vi "GetData.vi"(8 "error in (no error)":errorcluster, 10 "Channel":u8, 11 "ID In":i32) -> (0 "error out":errorcluster, 1 "Data information":T2 {"NbCols" min=5 max=7}, 2 "Current values":T1 {"EceRangeMax" format="%.2e"; "EceRangeMin" format="%.2e"; "EweRangeMax" format="%.2e"; "EweRangeMin" format="%.2e"; "Ece" format="%.2e"; "Ewe" format="%.2e"; "I" format="%.2e"; "TimeBase" format="%.2e"}, 3 "ID Out":i32, 4 "row2":u32[](array[numeric]), 5 "Data":dbl[][](array[numeric]), 6 "row3":u32[](array[numeric]), 7 "row4":u32[](array[numeric]))   [LabVIEW 2022 SP3, in "EClib functions.lvlib"]
doc: "Gets data from the selected channel."
uses:
  EClib functions.lvlib
  daff55f7-81b9-4493-b743-378d3d3ed068.vi
  68c41494-4949-413e-9d31-4f27a4ef7998.vi
  99021f18-7fd7-4697-be58-36819a2c27f0.vi
  61984fb0-cc5b-45ed-9757-d3fa5cda0840.vi
  fc0931df-71c6-4ee7-b843-224dab94ccff.vi
  daff55f7-81b9-4493-b743-378d3d3ed068.vi/7c5cbe08-cd9e-464e-aac1-cffdf31a2600.vi
  68c41494-4949-413e-9d31-4f27a4ef7998.vi/7c5cbe08-cd9e-464e-aac1-cffdf31a2600.vi
  99021f18-7fd7-4697-be58-36819a2c27f0.vi/db331072-caa1-433a-9332-c619978f86e3.vi
  61984fb0-cc5b-45ed-9757-d3fa5cda0840.vi/7c5cbe08-cd9e-464e-aac1-cffdf31a2600.vi
  fc0931df-71c6-4ee7-b843-224dab94ccff.vi/7c5cbe08-cd9e-464e-aac1-cffdf31a2600.vi
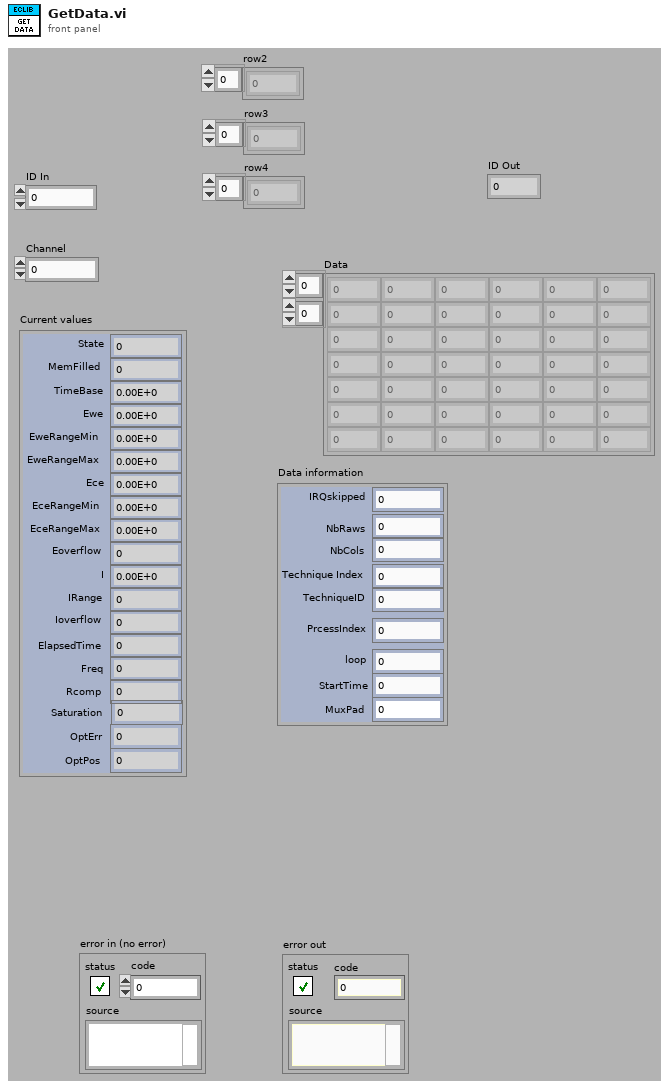
[diagram p1: front panel]
types:
  T1 = cluster{"State":i32, "MemFilled":i32, "TimeBase":sgl, " Ewe":sgl, " EweRangeMin":sgl, " EweRangeMax":sgl, "Ece":sgl, "EceRangeMin":sgl, "EceRangeMax":sgl, "Eoverflow":i32, "I":sgl, "IRange":i32, "Ioverflow":i32, "ElapsedTime":sgl, "Freq":sgl, "Rcomp":sgl, "Saturation":sgl, "OptErr":i32, "OptPos":i32}
  T2 = cluster{"IRQskipped":i32, "NbRaws":i32, "NbCols":i32, "Technique Index":i32, "TechniqueID":i32, "PrcessIndex":i32, "loop":i32, "StartTime":dbl, "MuxPad":i32}
  T3 = enum16{"unknown", "essential", "premium", "premium digicore"}
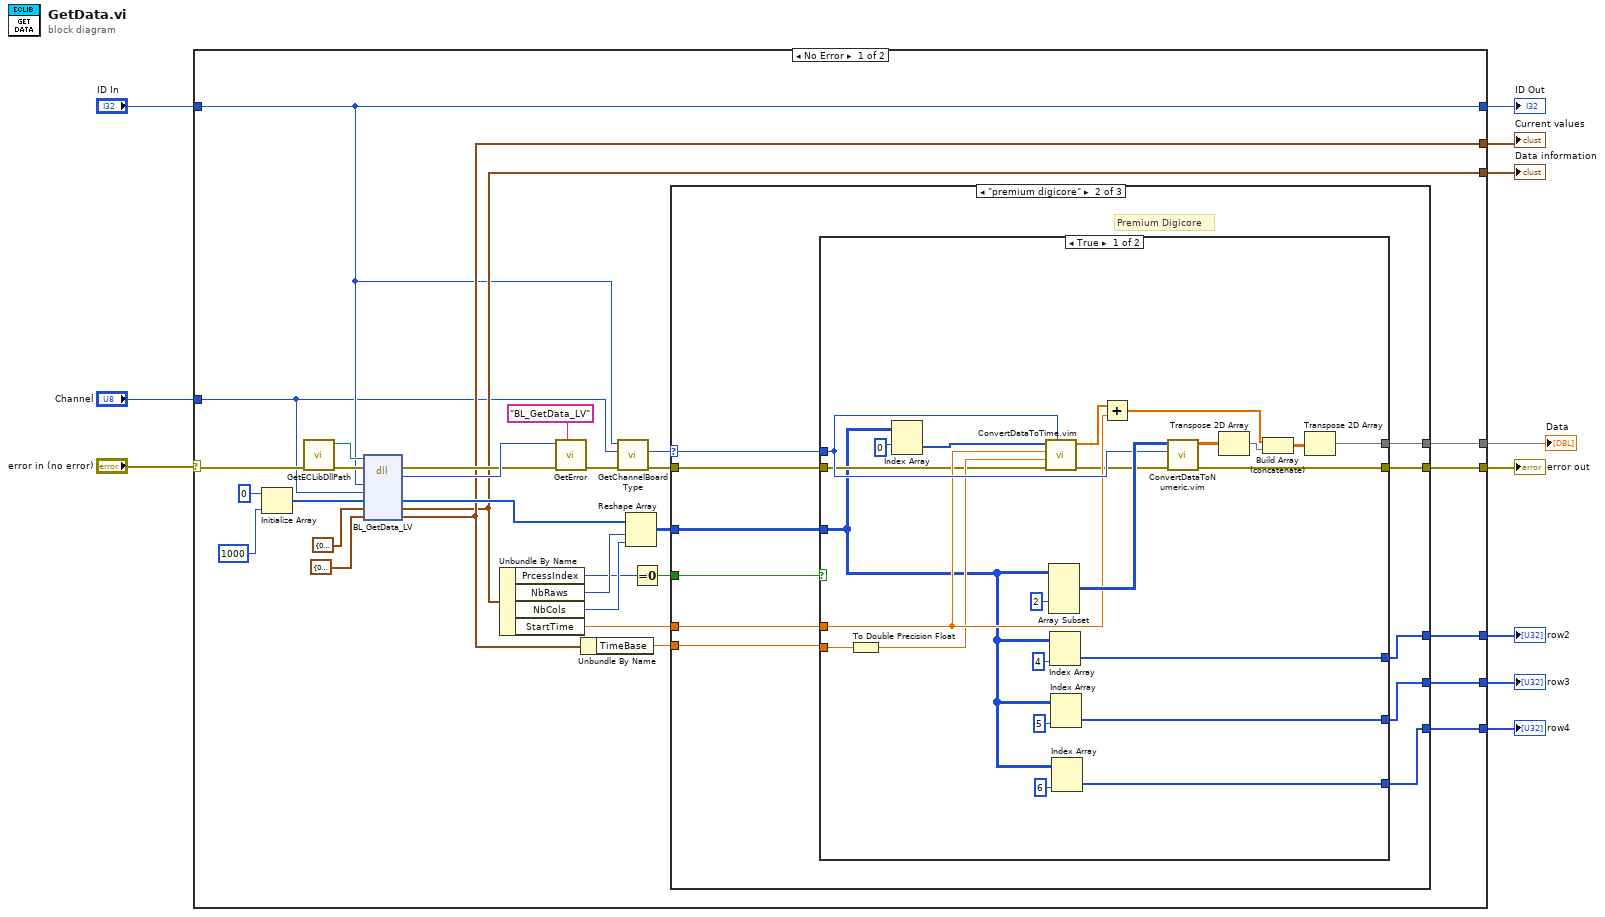
[diagram p0: block diagram]
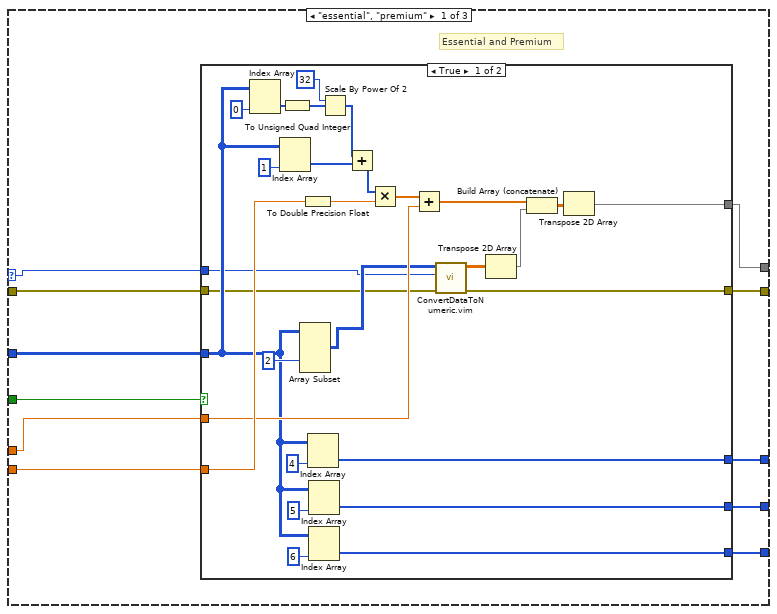
[diagram p2: hidden frame]
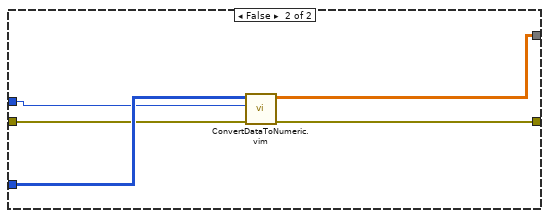
[diagram p3: hidden frame]
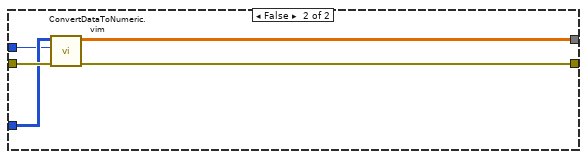
[diagram p4: hidden frame]
diagram:
  n1 = case shown="No Error" "error in (no error)" {
    selector: "error in (no error)" -> [w27 w130]
    tunnel: [w39 w130] -> w11
    tunnel: "ID In" -> [w13 w129]
    tunnel: "Channel" -> [w12 _]
    tunnel: [w23 _] -> w7
    tunnel: [w22 _] -> w6
    tunnel: [w20 _] -> w5
    tunnel: [w13 w129] -> w4
    tunnel: [w19 _] -> w3
    tunnel: [w18 _] -> w2
    tunnel: [w17 _] -> w1
    frame No Error {
      n2 = Initialize Array(u32 0 ("paramètre d'entrée"), 1000 ("dimension size")) -> (w41:u32[])
      n3 = call "GetECLibDllPath.vi"("error in (no error)"=w27) -> ("error out"=w25:errorcluster, "ECLibDLLPath"=w21:path)  [unwired: 9 in]
      n4 = dll-call lib="?" fn="BL_GetData_LV"(path in=w21, error in=w25, "arg1"=w13, "arg2"=w12, "arg3"=w41, "arg4"=T2 {"IRQskipped"=0, "NbRaws"=0, "NbCols"=0, "Technique Index"=0, "TechniqueID"=0, "PrcessIndex"=0, "loop"=0, "StartTime"=0.0, "MuxPad"=0} ("Data information"), "arg5"=T1 {"State"=0, "MemFilled"=0, "TimeBase"=0.0, " Ewe"=0.0, " EweRangeMin"=0.0, " EweRangeMax"=0.0, "Ece"=0.0, "EceRangeMin"=0.0, "EceRangeMax"=0.0, "Eoverflow"=0, "I"=0.0, "IRange"=0, "Ioverflow"=0, "ElapsedTime"=0.0, "Freq"=0.0, "Rcomp"=0.0, "Saturation"=0.0, "OptErr"=0, "OptPos"=0} ("Current values")) -> (error out=w24:errorcluster, "return type"=w26:i32, "arg3"=w38:u32[], "arg4"=w22:T2, "arg5"=w23:T1)  [unwired: 3 in, 1 out]
      n5 = Unbundle By Name(w22) -> ("PrcessIndex"=w33:i32, "NbRaws"=w37:i32, "NbCols"=w36:i32, "StartTime"=w32:dbl)
      n6 = call "GetError.vi"("DLLFunction"="BL_GetData_LV", "error in"=w24, "code"=w26) -> ("error out"=w15:errorcluster)  [unwired: 8 in]
      n7 = Unbundle By Name(w23) -> ("TimeBase"=w31:sgl)
      n8 = call "GetChannelBoardType.vi"("error in (no error)"=w15, "Channel"=w12, "ConnectionID IN"=w13) -> ("error out"=w14:errorcluster, "BoardType"=w16:T3)  [unwired: 5 in, 2 out]
      n9 = Reshape Array(w38, w37, w36) -> (w35:u32[][])
      n10 = Equal To 0?(x=w33) -> (x = 0?=w34:bool)
      n11 = case shown="\"premium digicore\"" w16 {
        selector: w16 -> [w44 w89 _]
        tunnel: [w48 w98 w128] -> w39
        tunnel: w35 -> [w53 w97 _]
        tunnel: w34 -> [w52 w96 _]
        tunnel: w32 -> [w51 w95 _]
        tunnel: w31 -> [w50 w94 _]
        tunnel: w14 -> [w43 w90 w128]
        tunnel: [w49 w93 _] -> w20
        tunnel: [w47 w92 _] -> w19
        tunnel: [w46 w91 _] -> w18
        tunnel: [w45 w88 _] -> w17
        frame "essential", "premium" {
          # "Essential and Premium"
          n12 = case shown="True" w52 {
            tunnel: w50 -> [w75 _]
            tunnel: w51 -> [w72 _]
            tunnel: [w66 w83] -> w49
            tunnel: w43 -> [w56 w85]
            tunnel: [w55 w84] -> w48
            tunnel: w53 -> [w59 w87]
            tunnel: [w65 _] -> w47
            tunnel: [w62 _] -> w46
            tunnel: [w61 _] -> w45
            tunnel: w44 -> [w57 w86]
            frame True {
              n13 = Index Array(array=w59, index (col)=0 ("indice désactivé (col)")) -> (element=w80:u32[])  [unwired: 1 in]
              n14 = Index Array(array=w59, index (col)=1 ("indice désactivé (col)")) -> (element=w76:u32[])  [unwired: 1 in]
              n15 = To Unsigned Quad Integer(1:w80) -> (0:w78:u64[])
              n16 = Array Subset(array=w59, index (col)=2 ("length")) -> (w58:u32[][])  [unwired: 3 in]
              n17 = To Double Precision Float(number=w75) -> (double precision float=w73:dbl)
              n18 = Index Array(array=w59, index (col)=4 ("disabled index (col)")) -> (element=w65:u32[])  [unwired: 1 in]
              n19 = Index Array(array=w59, index (col)=5 ("disabled index (col)")) -> (element=w62:u32[])  [unwired: 1 in]
              n20 = Index Array(array=w59, index (col)=6 ("disabled index (col)")) -> (element=w61:u32[])  [unwired: 1 in]
              n21 = Scale By Power Of 2(n=i16 32, x=w78) -> (x*2^n=w77:u64[])
              n22 = Add(x=w77, y=w76) -> (x+y=w74:u64[])
              n23 = Multiply(x=w74, y=w73) -> (x*y=w71:dbl[])
              n24 = Add(x=w71, y=w72) -> (x+y=w69:dbl[])
              n25 = call "ConvertDataToNumeric.vim"("error in (no error)"=w56, "BoardType"=w57, "Data"=w58) -> ("error out"=w55:errorcluster, "ConvertedTime"=w54:sgl[][])  [unwired: 7 in]
              n26 = Transpose 2D Array(2D array=w54) -> (transposed array=w68:sgl[][])
              n27 = Build Array (concatenate)(w69, w68) -> (w70:dbl[][])
              n28 = Transpose 2D Array(2D array=w70) -> (transposed array=w66:dbl[][])
            }
            frame False {
              n29 = call "ConvertDataToNumeric.vim"("error in (no error)"=w85, "BoardType"=w86, "Data"=w87) -> ("error out"=w84:errorcluster, "ConvertedTime"=w83:sgl[][])  [unwired: 7 in]
            }
          }
        }
        frame "premium digicore" {
          # "Premium Digicore"
          n30 = case shown="True" w96 {
            tunnel: w94 -> [w112 _]
            tunnel: w95 -> [w106 _]
            tunnel: [w117 w125] -> w93
            tunnel: w90 -> [w103 w127]
            tunnel: [w109 w124] -> w98
            tunnel: w97 -> [w100 w126]
            tunnel: [w116 _] -> w92
            tunnel: [w113 _] -> w91
            tunnel: w89 -> [w108 w123]
            tunnel: [w99 _] -> w88
            frame True {
              n31 = To Double Precision Float(number=w112) -> (double precision float=w105:dbl)
              n32 = Index Array(array=w100, index (col)=0 ("indice désactivé (col)")) -> (element=w107:u32[])  [unwired: 1 in]
              n33 = call "ConvertDataToTime.vim"("BoardType"=w108, "error in (no error)"=w103, "Timebase"=w105, "StartTime"=w106, "Data"=w107) -> ("error out"=w102:errorcluster, "ConvertedTime"=w104:dbl[])  [unwired: 5 in]
              n34 = Array Subset(array=w100, index (col)=2 ("length")) -> (w111:u32[][])  [unwired: 3 in]
              n35 = Index Array(array=w100, index (col)=4 ("disabled index (col)")) -> (element=w116:u32[])  [unwired: 1 in]
              n36 = Index Array(array=w100, index (col)=5 ("disabled index (col)")) -> (element=w113:u32[])  [unwired: 1 in]
              n37 = Index Array(array=w100, index (col)=6 ("disabled index (col)")) -> (element=w99:u32[])  [unwired: 1 in]
              n38 = Add(x=w104, y=w106) -> (x+y=w120:dbl[])
              n39 = call "ConvertDataToNumeric.vim"("error in (no error)"=w102, "BoardType"=w108, "Data"=w111) -> ("error out"=w109:errorcluster, "ConvertedTime"=w110:sgl[][])  [unwired: 7 in]
              n40 = Transpose 2D Array(2D array=w110) -> (transposed array=w119:sgl[][])
              n41 = Build Array (concatenate)(w120, w119) -> (w121:dbl[][])
              n42 = Transpose 2D Array(2D array=w121) -> (transposed array=w117:dbl[][])
            }
            frame False {
              n43 = call "ConvertDataToNumeric.vim"("error in (no error)"=w127, "BoardType"=w123, "Data"=w126) -> ("error out"=w124:errorcluster, "ConvertedTime"=w125:sgl[][])  [unwired: 7 in]
            }
          }
        }
        frame "unknown" {
        }
      }
    }
    frame Error {
    }
  }
  "error out" <- w11
  "Current values" <- w7
  "Data information" <- w6
  "Data" <- w5
  "ID Out" <- w4
  "row2" <- w3
  "row3" <- w2
  "row4" <- w1
